vi "Write writeRDs.vi"(8 "error in":errorcluster, 10 "Write?":bool, 11 "CRDS in":refnum<class "CRDS.lvclass">) -> (0 "error out":errorcluster, 3 "CRDS out":refnum<class "CRDS.lvclass">)   [LabVIEW 2015, in "CRDS.lvclass"]
uses:
  CRDS.lvclass
  Session Log/System Log.lvclass
  File IO/Class/File Observer.lvclass
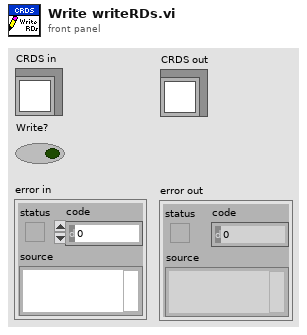
[diagram p1: front panel]
types:
  T1 = typedef "Session - Root.lvclass/Session Handle.ctl" = refnum<data-value>
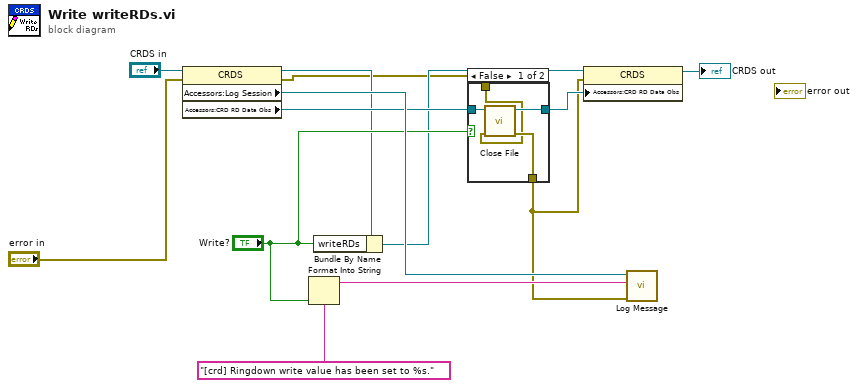
[diagram p0: block diagram]
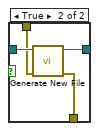
[diagram p2: hidden frame]
diagram:
  n1 = property class="CRDS"(reference="CRDS in", error in="error in") -> (reference out=w4:refnum<class "CRDS.lvclass">, error out=w2:errorcluster, "Accessors:Log Session"=w9:T1, "Accessors:CRD RD Data Obs"=w7:refnum<class "File Observer.lvclass">)
  n2 = Format Into String(format string="[crd] Ringdown write value has been set to %s.", "Write?") -> (resulting string=w10:string)  [unwired: 2 in, 1 out]
  n3 = Bundle By Name(cluster=w4, "writeRDs"="Write?") -> (w3:refnum<class "CRDS.lvclass">)
  n4 = case shown="False" "Write?" {
    tunnel: w7 -> [w17 w21]
    tunnel: [w16 w20] -> w5
    tunnel: w2 -> [w14 w19]
    tunnel: [w15 w18] -> w1
    frame False {
      n5 = call-dynamic "Close File.vi"("error in"=w14, "File Obs in"=w17) -> ("error out"=w15:errorcluster, "File Obs out"=w16:refnum<class "File Observer.lvclass">)  [unwired: 8 in]
    }
    frame True {
      n6 = call-dynamic "Generate New File.vi"("error in"=w19, "File Obs in"=w21) -> ("error out"=w18:errorcluster, "File Obs out"=w20:refnum<class "File Observer.lvclass">)  [unwired: 7 in, 1 out]
    }
  }
  n7 = property class="CRDS"(reference=w3, error in=w1, "Accessors:CRD RD Data Obs"=w5) -> (reference out=→"CRDS out":refnum<class "CRDS.lvclass">)  [unwired: 1 out]
  n8 = call "Log Message.vi"("error in"=w1, "MSG In"=w10, "session in"=w9) -> ()  [unwired: 7 in, 2 out]
